vi "Datos In.vi"() -> ()   [LabVIEW 2019]
panel:
  out "Datos In":T1
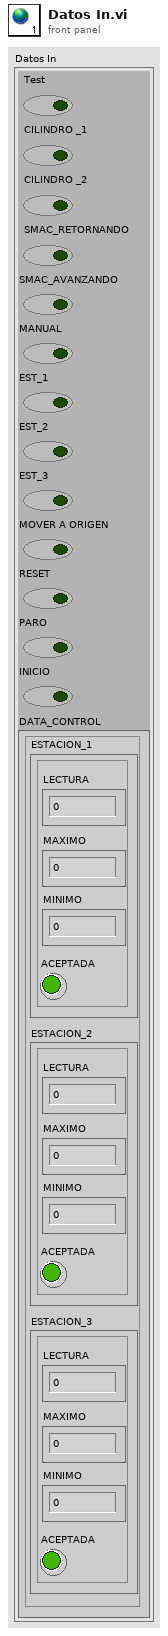
[diagram p1: front panel]
types:
  T1 = cluster{"Test":bool, "CILINDRO _1":bool, "CILINDRO _2":bool, "SMAC_RETORNANDO":bool, "SMAC_AVANZANDO":bool, "MANUAL":bool, "EST_1":bool, "EST_2":bool, "EST_3":bool, "MOVER A ORIGEN":bool, "RESET":bool, "PARO":bool, "INICIO":bool, "DATA_CONTROL":cluster{"ESTACION_1":cluster{"ACEPTADA":bool, "MAXIMO":dbl, "MINIMO":dbl, "LECTURA":dbl}, "ESTACION_2":cluster{"ACEPTADA":bool, "MAXIMO":dbl, "MINIMO":dbl, "LECTURA":dbl}, "ESTACION_3":cluster{"ACEPTADA":bool, "MAXIMO":dbl, "MINIMO":dbl, "LECTURA":dbl}}}
diagram:
